vi "Upgrade dotNET Socket to SSL.vi"(8 "error in (no error)":errorcluster, 11 "Socket in":refnum<class "Socket.lvclass">) -> (0 "error out":errorcluster, 3 "dotNET SSL Socket out":refnum<class "dotNET SSL Server.lvclass">)   [LabVIEW 2013, in "dotNET SSL Socket.lvlib" / "dotNET SSL Server.lvclass"]
doc: "Upgrades a dotNET Socket (from the dotNET Listener VIs) to an SSL Server connection. After calling this VI, the SSL should be configured and then the Handshake VI called."
uses:
  dotNET SSL Server.lvclass
  <vilib>/MediaMongrels Ltd/WebSockets/Sockets/Socket/Socket.lvclass
  dotNET TCP Socket/dotNET TCP Socket.lvclass
  dotNET TCP Socket/dotNET TCP Socket.lvclass/dotNET TCP Socket.ctl
  Z:/LabVIEW Working Directory/MediaMongrels Library Packages/secure-websockets-addon/Source/dotNET SSL Socket/TimeoutSSLStream.dll
  TimeoutSSLStream.dll
  dotNET SSL Socket/dotNET SSL Socket.lvclass/dotNET SSL Socket.ctl
  dotNET TCP Socket/Read TcpClient.vi
  dotNET SSL Socket/Write SSLStream.vi
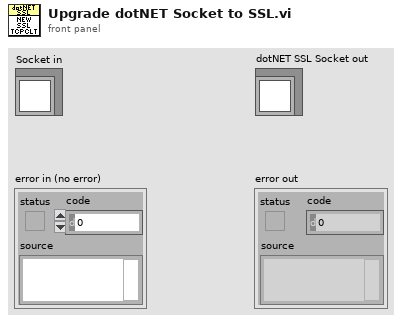
[diagram p1: front panel]
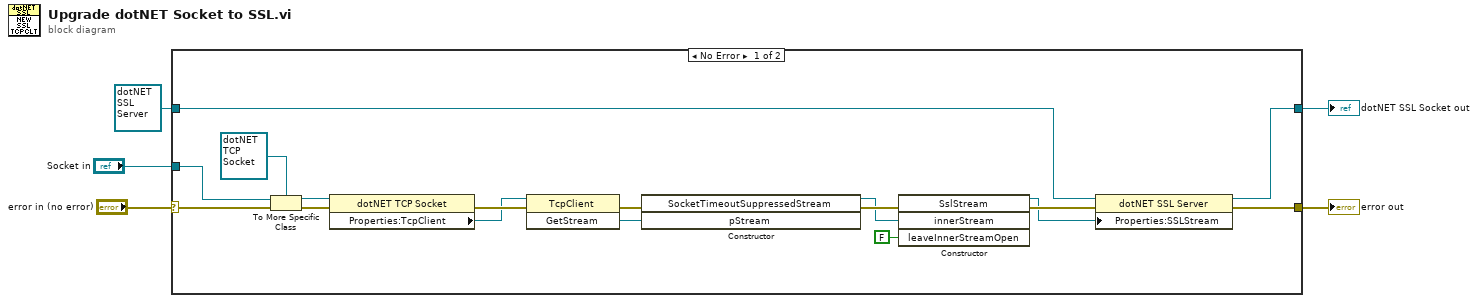
[diagram p0: block diagram]
diagram:
  n1 = case shown="No Error" "error in (no error)" {
    selector: "error in (no error)" -> [w19 w23]
    tunnel: [w17 w23] -> w4
    tunnel: [w15 w22] -> w2
    tunnel: refnum<class "dotNET SSL Server.lvclass"> refnum ("dotNET SSL Socket in") -> [w16 w22]
    tunnel: "Socket in" -> [w13 _]
    frame No Error {
      n2 = To More Specific Class(target class=refnum<class "dotNET TCP Socket.lvclass"> refnum ("dotNET SSL Socket.lvlib:dotNET TCP Socket.lvclass"), reference=w13, error in=w19) -> (specific class reference=w10:refnum<class "dotNET TCP Socket.lvclass">, error out=w14:errorcluster)
      n3 = property class="dotNET TCP Socket"(reference=w10, error in=w14) -> (error out=w11:errorcluster, "Properties:TcpClient"=w9:refnum<k24>)  [unwired: 1 out]
      n4 = invoke class="TcpClient" method="GetStream"(reference=w9, error in=w11) -> (error out=w8:errorcluster, "GetStream"=w7:refnum<k24>)  [unwired: 1 in, 1 out]
      n5 = constructor class="SocketTimeoutSuppressedStream"(error in=w8, "pStream"=w7) -> (reference out=w6:refnum<k24>)  [unwired: 2 in, 3 out]
      n6 = constructor class="SslStream"(error in=w8, "innerStream"=w6, "leaveInnerStreamOpen"=FALSE) -> (reference out=w18:refnum<k24>, error out=w20:errorcluster)  [unwired: 2 in, 3 out]
      n7 = property class="dotNET SSL Server"(reference=w16, error in=w20, "Properties:SSLStream"=w18) -> (reference out=w15:refnum<class "dotNET SSL Server.lvclass">, error out=w17:errorcluster)
    }
    frame Error {
    }
  }
  "error out" <- w4
  "dotNET SSL Socket out" <- w2
